vi "HDF5_Write_TimeDomain_Record_20181120_b.vi"(0 "ToneRefs":T1 {"Group_ref" format="%.0x"; "Cal"."Downshift_dset" format="%.0x"; "Cal"."DeltaPhase_dset" format="%.0x"; "Cal"."Phase_dset" format="%.0x"; "Cal"."SNR_dset" format="%.0x"; "Cal"."df_dset" format="%.0x"; "Cal"."PeakLoc_dset" format="%.0x"; "Cal"."MaxValue_dset" format="%.0x"; "Cal"."TImeStamp_dset" format="%.0x"; "Cal"."TimeString_dset" format="%.0x"; "Beac"."Downshift_dset" format="%.0x"; "Beac"."DeltaPhase_dset" format="%.0x"; "Beac"."Phase_dset" format="%.0x"; "Beac"."SNR_dset" format="%.0x"; "Beac"."df_dset" format="%.0x"; "Beac"."PeakLoc_dset" format="%.0x"; "Beac"."MaxValue_dset" format="%.0x"; "Beac"."TImeStamp_dset" format="%.0x"; "Beac"."TimeString_dset" format="%.0x"; "CalZoom_dSet" format="%.0x"; "BeacZoom_dSet" format="%.0x"}, 5 "TimeDomain":T4, 11 "error in":errorcluster) -> (15 "error out":errorcluster)   [LabVIEW 2018]
doc: "Write a single Tone<x> record with timestamp:\nTone1\n Beac - cluster\n BeacZoom - 1024 element Double array (waveform) \n Cal - cluster\n CalZoom - 1024 element Double array (waveform)"
uses:
  Controls/Enums/TargetNumber.ctl
  Controls/Clusts/TimeDomainData.ctl
  HDF5_Tone_refs.ctl
  Controls/Clusts/ToneGroupRefsClust.ctl
  <vilib>/addons/h5labview2/base/hid_t.ctl
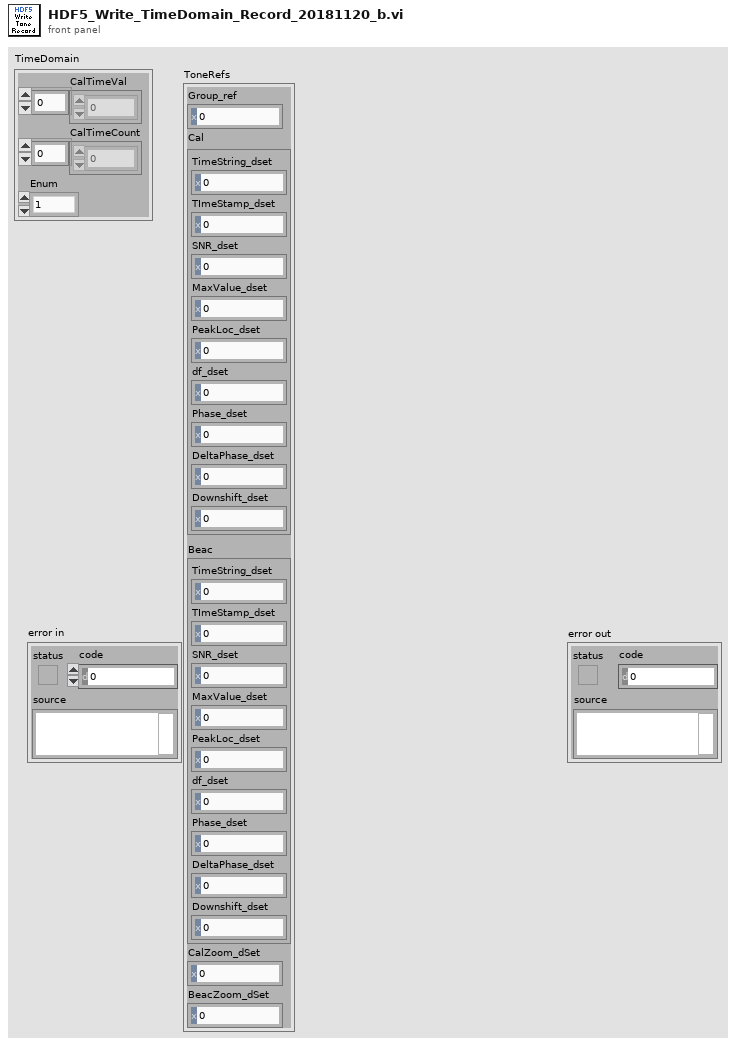
[diagram p1: front panel]
types:
  T1 = typedef "ToneGroupRefsClust.ctl" = cluster{"Group_ref":T2, "Cal":T3, "Beac":T3, "CalZoom_dSet":T2, "BeacZoom_dSet":T2}
  T2 = typedef "hid_t.ctl" = i32
  T3 = typedef "HDF5_Tone_refs.ctl" = cluster{"TimeString_dset":T2, "TImeStamp_dset":T2, "SNR_dset":T2, "MaxValue_dset":T2, "PeakLoc_dset":T2, "df_dset":T2, "Phase_dset":T2, "DeltaPhase_dset":T2, "Downshift_dset":T2}
  T4 = typedef "TimeDomainData.ctl" = cluster{"CalTimeVal":dbl[], "CalTimeCount":u32[], "Enum":T5}
  T5 = typedef "TargetNumber.ctl" = enum16{"1", "2", "3", "4"}
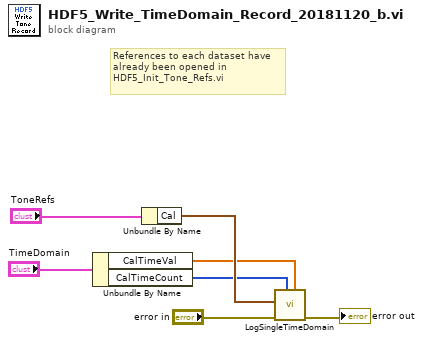
[diagram p0: block diagram]
diagram:
  # "References to each dataset have \nalready been opened in \nHDF5_Init_Tone_Refs.vi"
  n1 = Unbundle By Name("TimeDomain") -> ("CalTimeVal"=w3:dbl[], "CalTimeCount"=w4:u32[])
  n2 = Unbundle By Name("ToneRefs") -> ("Cal"=w6:T3)
  n3 = call "LogSingleTimeDomain.vi"("TimeDomainVal"=w3, "TimeDomainCount"=w4, "error in"="error in", "Cal"=w6) -> ("error out"=→"error out":errorcluster)  [unwired: 7 in]
